vi "PH_ImageOperator.get Cam Settings.vi"(0 "i ref in":refnum<vi>, 2 "Cam Settings":T1={"Cam ID"="N/A", "Gain"=nan, "Brightness"=nan, "Shutter"=nan, "Mode"=-1}, 3 "Cam Info Failure":bool, 5 "error in (no error)":errorcluster) -> (14 "i ref out":refnum<vi>, 19 "error out":errorcluster)   [LabVIEW 2014, in "PH_ImageOperator.lvlib"]
doc: "This VI stores the incoming information to own attributes."
uses:
  PH_ImageOperator.lvlib
  PH_Basics/PH_Cam_BaseClass/PH_Cam_BaseClass.Settings.ctl
  PH_Basics/PH_Img_BaseClass/PH_Img_BaseClass.lvlib
  PH_Basics/PH_Cam_BaseClass/PH_Cam_BaseClass.lvlib
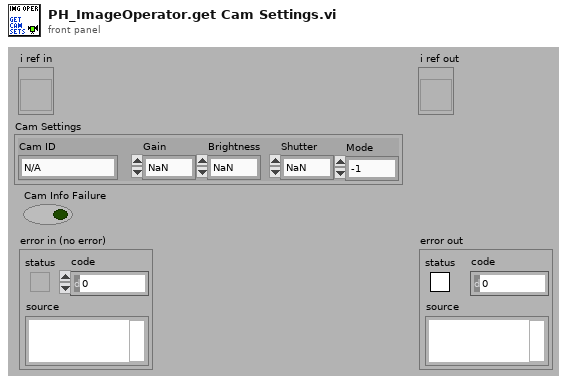
[diagram p1: front panel]
types:
  T1 = typedef "PH_Cam_BaseClass.lvlib/PH_Cam_BaseClass.Settings.ctl" = cluster{"Cam ID":string, "Gain":dbl, "Brightness":dbl, "Shutter":dbl, "Mode":i32}
  T2 = cluster{"Cam ID":string, "Gain":dbl, "Brightness":dbl, "Shutter":dbl, "Cam Error":bool, "Mode":i32}
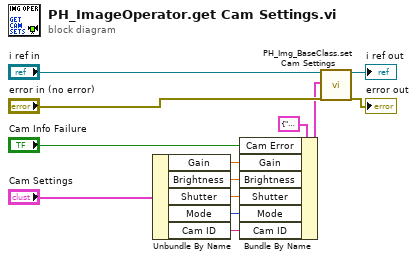
[diagram p0: block diagram]
diagram:
  n1 = Unbundle By Name("Cam Settings") -> ("Gain"=w10:dbl, "Brightness"=w9:dbl, "Shutter"=w8:dbl, "Mode"=w7:i32, "Cam ID"=w6:string)
  n2 = Bundle By Name(cluster=T2 {"Cam ID"="N/A", "Gain"=nan, "Brightness"=nan, "Shutter"=nan, "Cam Error"=TRUE, "Mode"=-1} ("Cam Settings"), "Cam Error"="Cam Info Failure", "Gain"=w10, "Brightness"=w9, "Shutter"=w8, "Mode"=w7, "Cam ID"=w6) -> (w1:T2)
  n3 = call "PH_Img_BaseClass.set Cam Settings.vi"("i ref in"="i ref in", "Cam Settings"=w1, "error in (no error)"="error in (no error)") -> ("i ref out"=→"i ref out":refnum<vi>, "error out"=→"error out":errorcluster)  [unwired: 15 in]
